vi "ListAvailablePackagesInFeed.vi"(8 "Error In":errorcluster, 10 "Log File Path":path, 11 "FeedURL(s)":string="https://download.ni.com/support/nipkg/products/ni-t/ni-teststand-2020/20.0/released") -> (0 "Error Out":errorcluster)   [LabVIEW 2019, in "CEPM.lvlib"]
uses:
  CEPM.lvlib
  Typedefs/PackageMeta.ctl
  <vilib>/SLL Toolkit/SLL File IO/Spreadsheet/CSV Logger/_Typedefs/String Key Value Pair Cluster.ctl
  <vilib>/SLL Toolkit/SLL File IO/Spreadsheet/CSV Logger/SLL CSV Logger.lvclass
panel:
  out "PackageMeta":T1[](array[typedef])
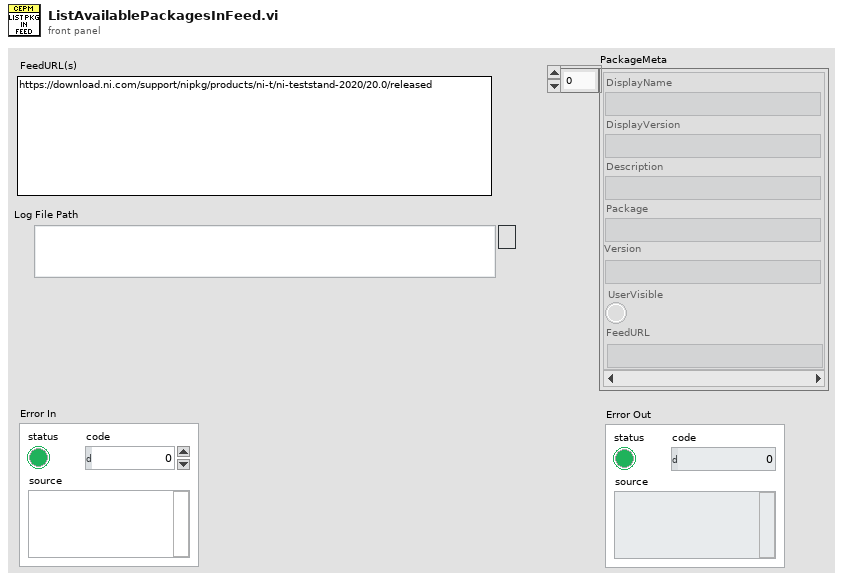
[diagram p1: front panel]
types:
  T1 = typedef "CEPM.lvlib/PackageMeta.ctl" = cluster{"DisplayName":string, "DisplayVersion":string, "Description":string, "Package":string, "Version":string, "UserVisible":bool, "FeedURL":string}
  T2 = typedef "SLL Spreadsheet.lvlib/SLL CSV Logger.lvclass/String Key Value Pair Cluster.ctl" = cluster{"Key":string, "Value":string}
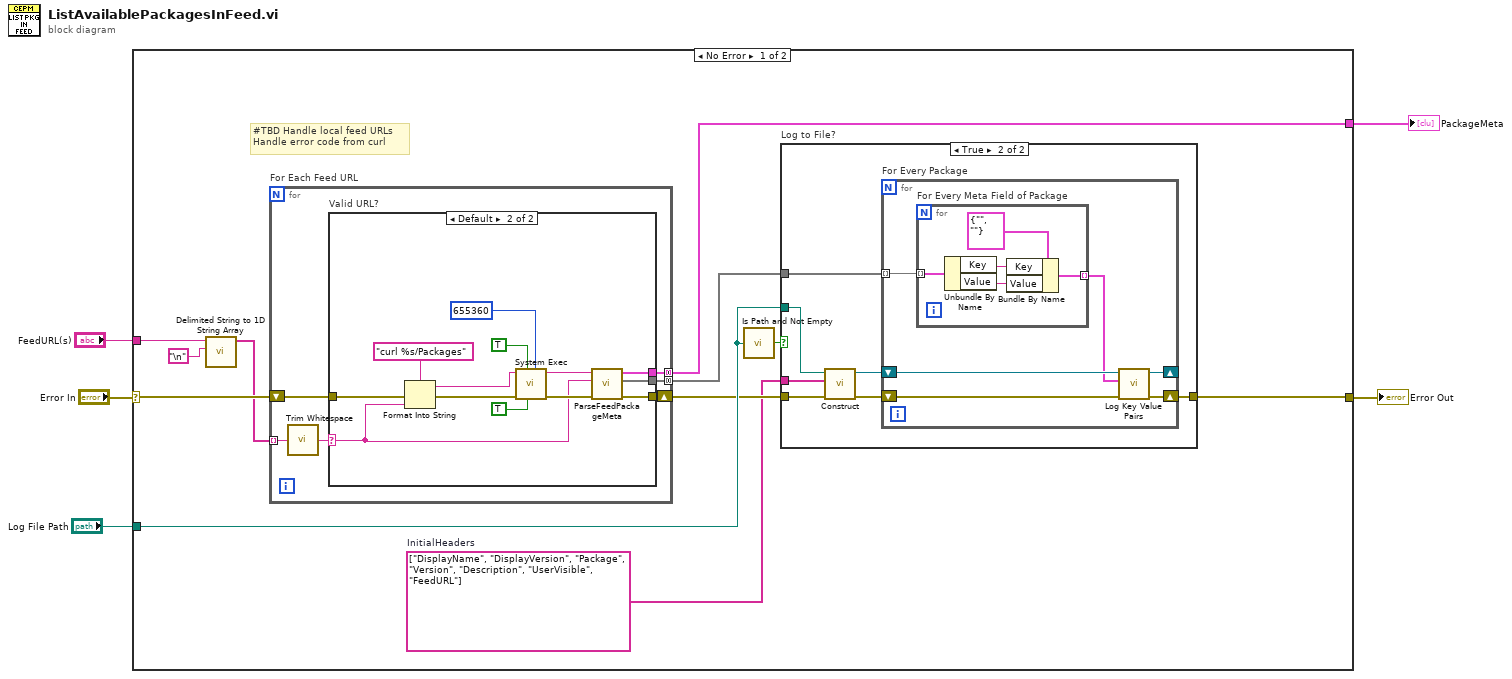
[diagram p0: block diagram]
diagram:
  n1 = case shown="No Error" "Error In" {
    selector: "Error In" -> [w16 w56]
    tunnel: [w10 w56] -> w4
    tunnel: "FeedURL(s)" -> [w8 _]
    tunnel: [w15 _] -> w2
    tunnel: "Log File Path" -> [w12 _]
    frame No Error {
      w9 = string[] ["DisplayName", "DisplayVersion", "Package", "Version", "Description", "UserVisible", "FeedURL"]  # InitialHeaders
      # "#TBD Handle local feed URLs\nHandle error code from curl"
      n2 = call <vilib>:"Delimited String to 1D String Array.vi"("delimiter"="\n", "delimited string"=w8) -> ("string array"=w6:string[])  [unwired: 9 in]
      n3 = for "For Each Feed URL" {
        tunnel: [w40] -> w15 mode=concatenating
        tunnel: [w39] -> w14 mode=concatenating
        shift-right: [w38] -> w11
        shift-left: w16 -> [w41]
        tunnel: w6 -> [w37] mode=indexing
        n4 = call <vilib>:"Trim Whitespace.vi"("string"=w37) -> ("trimmed string"=w36:string)  [unwired: 1 in]
        n5 = case "Valid URL?" shown="Default" w36 {
          selector: w36 -> [_ w43]
          tunnel: w41 -> [w42 w55]
          tunnel: [_ w46] -> w40
          tunnel: [_ w45] -> w39
          tunnel: [w42 w44] -> w38
          frame "" {
          }
          frame Default {
            n6 = Format Into String(format string="curl %s/Packages", error in=w55, w43) -> (resulting string=w52:string, error out=w54:errorcluster)  [unwired: 1 in]
            n7 = call <vilib>:"System Exec.vi"("expected output size  (4096)"=u32 655360, "run minimized? (F)"=TRUE, "wait until completion? (T)"=TRUE, "error in (no error)"=w54, "command line"=w52) -> ("error out"=w48:errorcluster, "standard output"=w47:string)  [unwired: 3 in, 2 out]
            n8 = call "ParseFeedPackageMeta.vi"("Error In"=w48, "FeedURL"=w43, "FeedPackageMeta"=w47) -> ("Error Out"=w44:errorcluster, "PackageMetaMap"=w45:map{string, string}[], "PackageMeta"=w46:T1[])  [unwired: 6 in]
          }
        }
      }
      n9 = call <vilib>:"Is Path and Not Empty.vi"("path"=w12) -> ("Is Path and Not Empty?"=w13:bool)  [unwired: 4 in]
      n10 = case "Log to File?" shown="True" w13 {
        tunnel: w14 -> [_ w24]
        tunnel: w12 -> [_ w23]
        tunnel: w11 -> [w17 w20]
        tunnel: [w17 w19] -> w10
        tunnel: w9 -> [_ w18]
        frame False {
        }
        frame True {
          n11 = call <vilib>:"Construct.vi"("error in (no error)"=w20, "Starter Headers[]"=w18, "File Path"=w23) -> ("error out"=w22:errorcluster, "SLL CSV Logger out"=w21:refnum<class "SLL CSV Logger.lvclass">)  [unwired: 7 in]
          n12 = for "For Every Package" {
            tunnel: w24 -> [w30] mode=indexing
            shift-right: [w25] -> w19
            shift-left: w22 -> [w26]
            shift-right: [w28] -> _
            shift-left: w21 -> [w29]
            n13 = for "For Every Meta Field of Package" {
              tunnel: w30 -> [w35] mode=indexing
              tunnel: [w31] -> w27 mode=indexing
              n14 = Unbundle By Name(w35) -> ("Key"=w33:string, "Value"=w32:string)
              n15 = Bundle By Name(cluster=T2 {"Key"="", "Value"=""} ("Cluster"), "Key"=w33, "Value"=w32) -> (w31:T2)
            }
            n16 = call <vilib>:"Log Key Value Pairs.vi"("error in (no error)"=w26, "String Key Value Pairs"=w27, "SLL Spreadsheet Logger in"=w29) -> ("error out"=w25:errorcluster, "SLL Spreadsheet Logger out"=w28:refnum<class "SLL CSV Logger.lvclass">)  [unwired: 7 in]
          }
        }
      }
    }
    frame Error {
    }
  }
  "Error Out" <- w4
  "PackageMeta" <- w2
